vi "AddToAccessList.vi"(8 "error in (no error)":errorcluster, 11 "VItoAdd":refnum<vi>) -> (0 "error out":errorcluster, 2 "Server:VI Access List":string[](array[string]))   [LabVIEW 2021]
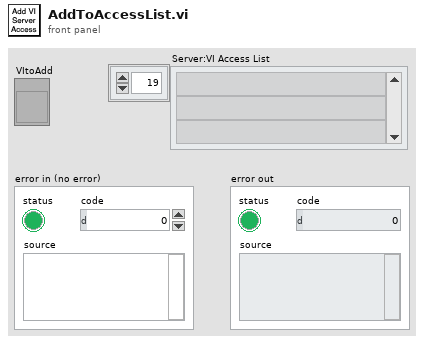
[diagram p1: front panel]
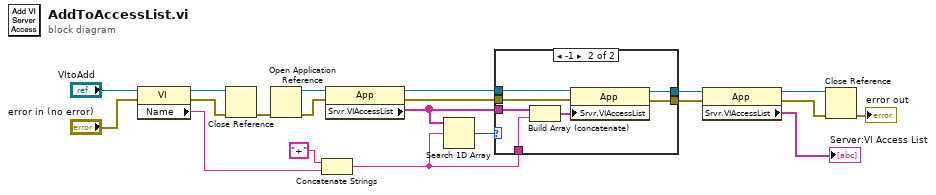
[diagram p0: block diagram]
diagram:
  n1 = property class="VI"(reference="VItoAdd", error in="error in (no error)") -> (reference out=w3:refnum<vi>, error out=w2:errorcluster, "Name"=w17:string)
  n2 = Close Reference(reference=w3, error in (no error)=w2) -> (error out=w1:errorcluster)
  n3 = Open Application Reference(8:w1) -> (0:w18:errorcluster, 3:w20:refnum<vi>)  [unwired: 3 in]
  n4 = Concatenate Strings("+" ("string"), w17) -> (w5:string)
  n5 = property class="App"(reference=w20, error in=w18) -> (reference out=w19:refnum<vi>, error out=w16:errorcluster, "Srvr.VIAccessList"=w6:string[])
  n6 = Search 1D Array(1D array=w6, element=w5) -> (index of element=w4:i32)  [unwired: 1 in]
  n7 = case shown="-1" w4 {
    tunnel: w19 -> [w22 w29]
    tunnel: w16 -> [w21 w27]
    tunnel: [w22 w26] -> w14
    tunnel: [w21 w25] -> w13
    tunnel: w6 -> [_ w24]
    tunnel: w5 -> [_ w23]
    frame 0, Default {
    }
    frame -1 {
      n8 = Build Array (concatenate)(w24, w23) -> (w28:string[])
      n9 = property class="App"(reference=w29, error in=w27, "Srvr.VIAccessList"=w28) -> (reference out=w26:refnum<vi>, error out=w25:errorcluster)
    }
  }
  n10 = property class="App"(reference=w14, error in=w13) -> (reference out=w12:refnum<vi>, error out=w11:errorcluster, "Srvr.VIAccessList"=→"Server:VI Access List":string[])
  n11 = Close Reference(reference=w12, error in (no error)=w11) -> (error out=→"error out":errorcluster)
